vi "Get Platform.vi"(8 "error in (no error)":errorcluster, 11 "PlatformArrayPanel in":refnum<class "PlatformArrayPanel.lvclass">) -> (0 "error out":errorcluster, 2 "Platform":refnum<class "Platform.lvclass">, 3 "PlatformArrayPanel out":refnum<class "PlatformArrayPanel.lvclass">)   [LabVIEW 2020, in "PicoG-App.lvlib" / "PlatformArrayPanel.lvclass"]
uses:
  PlatformArrayPanel.lvclass
  PlatformArrayPanel.lvclass/PlatformArrayPanel.ctl
  Builds/picoG/ppl/PicoG-Core.lvlibp/PicoG-Processor/PicoG-Core/DeployPlatform/Platform.lvclass
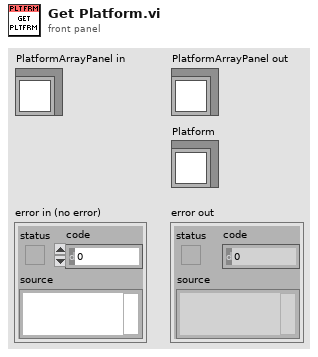
[diagram p1: front panel]
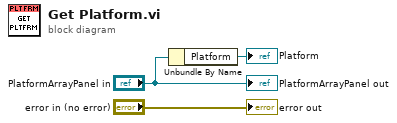
[diagram p0: block diagram]
diagram:
  n1 = Unbundle By Name("PlatformArrayPanel in") -> ("Platform"=→"Platform":refnum<class "Platform.lvclass">)
  "error out" <- "error in (no error)"
  "PlatformArrayPanel out" <- "PlatformArrayPanel in"
